vi "timming_array_to_digital_waveform.vi"(0 "resolution":i32=100, 1 "delay array":dbl[](array[numeric]) format="%#_6e", 2 "burst period":dbl, 3 "burst count":i32, 4 "Burst?":bool) -> (6 "digital waveform":digitalwaveform(waveform)={"t0"=timestamp(0 s since 1904-01-01), "dt"=0.0, "Y"={"transitions"=[], "data"=[]}, "error"={"status"=FALSE, "code"=37421928, "source"=""}}, 7 "size(s)":i32[](array[numeric]))   [LabVIEW 2011]
doc: "takes the timing info recieved from the DG645 Delay generator and transforms it into a digital waveform graph.\nMakes sure, all timings are setup in reference to t0!"
panel:
  out "delta t":dbl
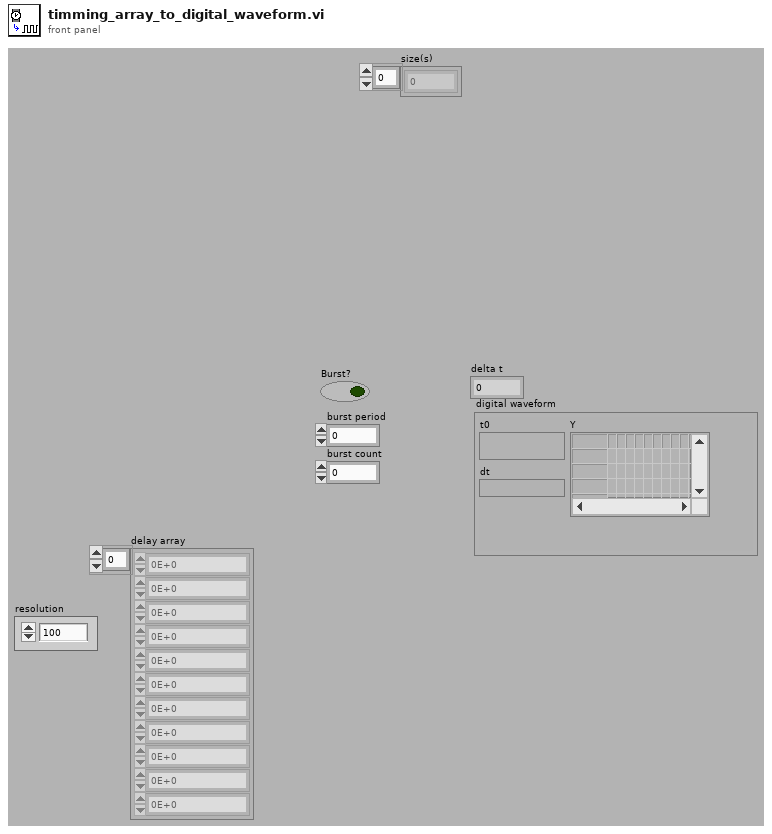
[diagram p1: front panel]
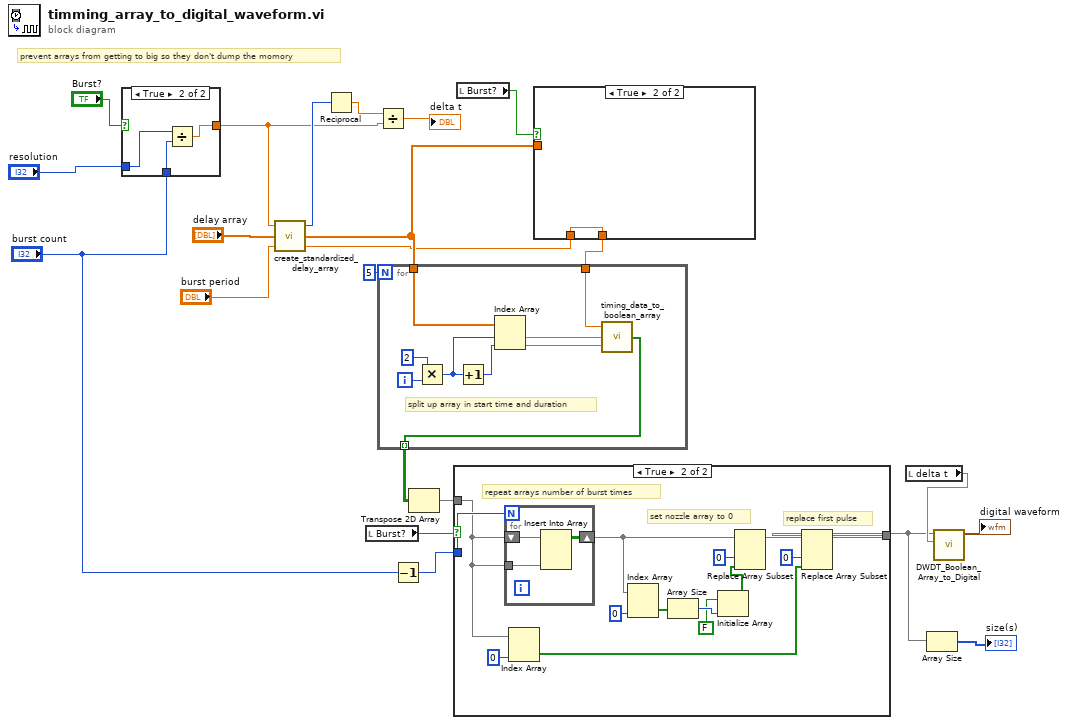
[diagram p0: block diagram]
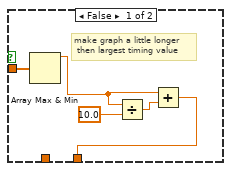
[diagram p4: hidden frame]
diagram:
  # "prevent arrays from getting to big so they don't dump the momory"
  n1 = case shown="True" "Burst?" {
    tunnel: [w23 w24] -> w8
    tunnel: "resolution" -> [w23 w26]
    tunnel: "burst count" -> [_ w25]
    frame False {
    }
    frame True {
      n2 = Divide(x=w26, y=w25) -> (x/y=w24:dbl)
    }
  }
  n3 = call "create_standardized_delay_array.vi"("burst period"="burst period", "delay array"="delay array", "resolution"=w8) -> ("corrected burst period"=w9:dbl, "standardize array"=w15:dbl[], "multiplier"=w16:i32)
  n4 = Reciprocal(x=w16) -> (1/x=w19:dbl)
  n5 = local read "Burst?"() -> (w14:bool)
  n6 = Divide(x=w19, y=w8) -> (x/y=→"delta t":dbl)
  n7 = Decrement(x="burst count") -> (x-1=w13:i32)
  n8 = local read "Burst?"() -> (w4:bool)
  n9 = case shown="True" w4 {
    tunnel: [w30 w32] -> w20
    tunnel: w15 -> [w27 _]
    tunnel: w9 -> [_ w32]
    frame False {
      # "make graph a little longer\n then largest timing value"
      n10 = Array Max & Min(array=w27) -> (max value=w28:dbl)  [unwired: 3 out]
      n11 = Divide(x=w28, y=10.0) -> (x/y=w29:dbl)
      n12 = Add(x=w28, y=w29) -> (x+y=w30:dbl)
    }
    frame True {
    }
  }
  n13 = for {
    N: 5 -> [_]
    tunnel: [w39] -> w21 mode=indexing
    tunnel: w20 -> [w38]
    tunnel: w15 -> [w33]
    i -> [w41]
    # "split up array in start time and duration"
    n14 = Multiply(x=2, y=w41) -> (x*y=w34:i32)
    n15 = Increment(x=w34) -> (x+1=w37:i32)
    n16 = Index Array(array=w33, index #1=w34, index #2=w37) -> (element #1=w36:dbl, element #2=w35:dbl)
    n17 = call "timing_data_to_boolean_array.vi"("end time [s]"=w35, "start time [s]"=w36, "overall length [s]"=w38) -> ("boolean timing array"=w39:bool[])  [unwired: 1 in]
  }
  n18 = Transpose 2D Array(2D array=w21) -> (transposed array=w17:bool[][])
  n19 = case shown="True" w14 {
    tunnel: w17 -> [w42 w45]
    tunnel: [w42 w47] -> w6
    tunnel: w13 -> [_ w56]
    frame False {
    }
    frame True {
      # "replace first pulse"
      # "repeat arrays number of burst times"
      # "set nozzle array to 0"
      n20 = for {
        N: w56 -> [_]
        shift-right: [w59] -> w52
        shift-left: w45 -> [w57]
        tunnel: w45 -> [w58]
        n21 = Insert Into Array(array=w57, new element=w58) -> (w59:bool[][])  [unwired: 2 in]
      }
      n22 = Index Array(array=w45, index (col)=0 ("disabled index (col)")) -> (element=w43:bool[])  [unwired: 1 in]
      n23 = Index Array(array=w52, index (col)=0 ("disabled index (col)")) -> (element=w54:bool[])  [unwired: 1 in]
      n24 = Array Size(array=w54) -> (size(s)=w55:i32)
      n25 = Initialize Array(FALSE, w55) -> (w51:bool[])
      n26 = Replace Array Subset(array=w52, new element=w51, index (col)=0 ("disabled index (col)")) -> (w48:bool[][])  [unwired: 1 in]
      n27 = Replace Array Subset(array=w48, new element=w43, index (col)=0 ("disabled index (col)")) -> (w47:bool[][])  [unwired: 1 in]
    }
  }
  n28 = local read "delta t"() -> (w12:dbl)
  n29 = Array Size(array=w6) -> (size(s)=→"size(s)":i32[])
  n30 = call "DWDT_Boolean_Array_to_Digital.vi"("delta t"=w12, "boolean array"=w6) -> ("digital waveform"=→"digital waveform":digitalwaveform)  [unwired: 8 in, 1 out]
